vi "Scratchpad.vi"() -> ()   [LabVIEW 2020, in "Test.lvlib"]
uses:
  Test.lvlib
  <vilib>/drjdpowell/SQLite Library/SQL Connection/Connection.lvclass
  <vilib>/drjdpowell/SQLite Library/SQLite.lvlib
  Conditum SQLite/SQLite/SQLite.lvclass
  <vilib>/IlluminatedG/IG Conditum/Conditum/Entity Manager/Entity Manager.lvclass
  User/User.lvclass
  User/Values.ctl
  <vilib>/IlluminatedG/IG Conditum/Conditum/Entity/Entity.lvclass
  <vilib>/drjdpowell/SQLite Library/SQL Connection/Open (string).vi
  <vilib>/drjdpowell/SQLite Library/SQL Connection/Execute SQL (No results).vi
  C:/Program Files (x86)/National Instruments/LabVIEW 2022/vi.lib/IlluminatedG/IG Conditum/Conditum/Entity/Entity.lvclass
  C:/dev/lv22CE/illuminated-g/lv-conditum-sqlite/Test/User/User.lvclass
  C:/Program Files (x86)/National Instruments/LabVIEW 2022/vi.lib/IlluminatedG/IG Conditum/Conditum/Database Platform/Database Platform.lvclass
  C:/dev/lv22CE/illuminated-g/lv-conditum-sqlite/Conditum SQLite/SQLite/SQLite.lvclass
  <vilib>/IlluminatedG/IG Conditum/Conditum/Entity ID.ctl
  <vilib>/IlluminatedG/IG Conditum/Conditum/Conditum.lvlib
panel:
  out "Time":dbl
  out "ID":T1
  out "error out":errorcluster
  in  "DB Path":path=path "C:/dev/lv/illuminated-g/lv-conditum-sqlite/Test/test.db"
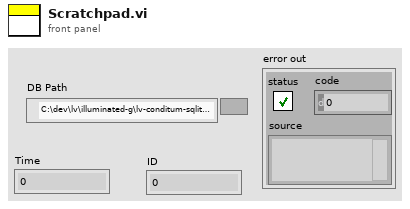
[diagram p1: front panel]
types:
  T1 = typedef "Conditum.lvlib/Entity ID.ctl" = i64
  T2 = typedef "Test.lvlib/User.lvclass/Values.ctl" = cluster{"Username":string, "Password":string, "Joined":timestamp, "Last Activity":timestamp, "Activated":bool, "Email":string, "Score":i64}
  T3 = enum16{"New or existing", "Existing", "Read only"}
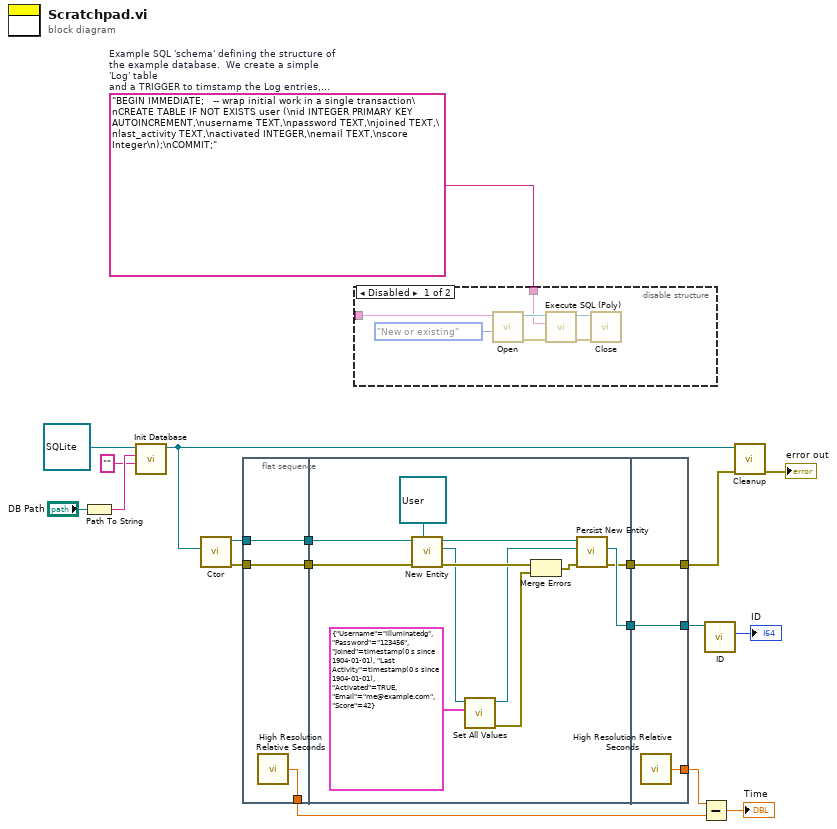
[diagram p0: block diagram]
diagram:
  w18 = "BEGIN IMMEDIATE;   -- wrap initial work in a single transaction\nCREATE TABLE IF NOT EXISTS user (\nid INTEGER PRIMARY KEY AUTOINCREMENT,\nusername TEXT,\npassword TEXT,\njoined TEXT,\nlast_activity TEXT,\nactivated INTEGER,\nemail TEXT,\nscore Integer\n);\nCOMMIT;"  # Example SQL 'schema' defining the structure of the example database.  We create a simple 'Log' table and a TRIGGER to timstamp the Log entries, then a simple 'Data' table
  n1 = Path To String(path="DB Path") -> (string=w17:string)
  n2 = call-dynamic "Init Database.vi"("Database"="", "Resource"=w17, "Database in"=refnum<class "SQLite.lvclass"> refnum) -> ("Database out"=w3:refnum<class "SQLite.lvclass">)  [unwired: 7 in, 1 out]
  n3 = call <vilib>:"Ctor.vi"("Database"=w3) -> ("error out"=w2:errorcluster, "Entity Manager out"=w1:refnum<class "Entity Manager.lvclass">)  [unwired: 9 in]
  n4 = flat-sequence {
    tunnel: w2 -> [w21]
    tunnel: w1 -> [w22]
    tunnel: [w22] -> w10
    tunnel: [w21] -> w9
    tunnel: [w20] -> w5
    tunnel: w10 -> [w33]
    tunnel: w9 -> [w32]
    tunnel: [w24] -> w8
    tunnel: [w23] -> w7
    tunnel: [w36] -> w12
    tunnel: [w37] -> w14
    tunnel: w8 -> [w37]
    tunnel: w7 -> [w36]
    tunnel: [w35] -> w6
    frame #0 {
      n5 = call <vilib>:"High Resolution Relative Seconds.vi"() -> ("relative seconds"=w20:dbl)
    }
    frame #1 {
      n6 = call <vilib>:"New Entity.vi"("Entity Type"=refnum<class "User.lvclass"> refnum ("Test.lvlib:User.lvclass"), "error in (no error)"=w32, "Entity Manager in"=w33) -> ("error out"=w34:errorcluster, "Entity"=w30:refnum<class "User.lvclass">, "Entity Manager out"=w27:refnum<class "Entity Manager.lvclass">)  [unwired: 6 in]
      n7 = call "Set All Values.vi"("Values"=T2 {"Username"="illuminatedg", "Password"="123456", "Joined"=timestamp(0 s since 1904-01-01), "Last Activity"=timestamp(0 s since 1904-01-01), "Activated"=TRUE, "Email"="me@example.com", "Score"=42}, "User in"=w30) -> ("error out"=w28:errorcluster, "User out"=w26:refnum<class "User.lvclass">)  [unwired: 8 in]
      n8 = Merge Errors(w34, w28) -> (w25:errorcluster)
      n9 = call <vilib>:"Persist New Entity.vi"("error in (no error)"=w25, "New Entity"=w26, "Entity Manager in"=w27) -> ("error out"=w23:errorcluster, "Entity"=w24:refnum<class "User.lvclass">)  [unwired: 6 in, 1 out]
    }
    frame #2 {
      n10 = call <vilib>:"High Resolution Relative Seconds.vi"() -> ("relative seconds"=w35:dbl)
    }
  }
  n11 = disable-structure shown="Disabled" {
    disable-tunnel: _ -> [w43 _]
    disable-tunnel: w18 -> [w40 _]
    frame Disabled {
      n12 = call-poly <vilib>:"Open.vi"("File Option"=T3."New or existing", "db file"=w43) -> ("error out"=w41:errorcluster, "SQLite Connection"=w44:refnum<class "Connection.lvclass">)  [unwired: 8 in]
      n13 = call-poly <vilib>:"Execute SQL (Poly).vi"("error in (no error)"=w41, "SQL"=w40, "SQLite Connection in"=w44) -> ("error out"=w39:errorcluster, "SQLite Connection"=w38:refnum<class "Connection.lvclass">)  [unwired: 7 in]
      n14 = call-dynamic "Close.vi"("error in (no error)"=w39, "SQLite Connection in"=w38) -> ()  [unwired: 9 in, 1 out]
    }
    frame Enabled {
    }
  }
  n15 = Subtract(x=w6, y=w5) -> (x-y=→"Time":dbl)
  n16 = call <vilib>:"ID.vi"("Entity in"=w14) -> ("ID"=→"ID":T1)  [unwired: 9 in, 1 out]
  n17 = call-dynamic "Cleanup.vi"("error in (no error)"=w12, "SQLite in"=w3) -> ("error out"=→"error out":errorcluster)  [unwired: 9 in]
